vi "Test 3.vi"() -> ()   [LabVIEW 2014, in "SetUp VIs.lvlib"]
uses:
  SetUp VIs.lvlib
panel:
  out "return count":u32
  out "error out 2":errorcluster
  out "error out":errorcluster
  out "read buffer":string
  in  "VISA resource name":refnum<visa-resource-name>
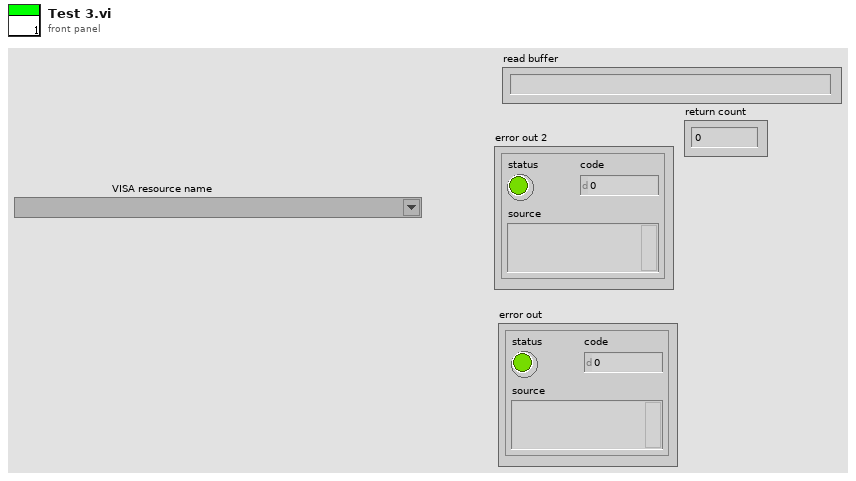
[diagram p1: front panel]
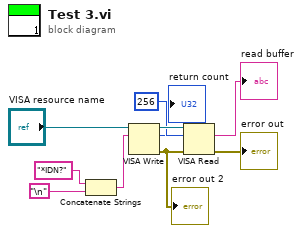
[diagram p0: block diagram]
diagram:
  n1 = Concatenate Strings("*IDN?" ("write buffer"), "\n") -> (w5:string)
  n2 = VISA Write(VISA resource name="VISA resource name", write buffer=w5) -> (VISA resource name out=w9:refnum<visa-resource-name>, return count=→"return count":u32, error out=w8:errorcluster)  [unwired: 1 in]
  "error out 2" <- w8
  n3 = VISA Read(VISA resource name=w9, byte count=u32 256, error in (no error)=w8) -> (read buffer=→"read buffer":string, error out=→"error out":errorcluster)  [unwired: 2 out]
